vi "VI Tree - error.vi"   [LabVIEW 2020]
uses:
  Filter Error Codes/Filter Error Codes (Array).vi
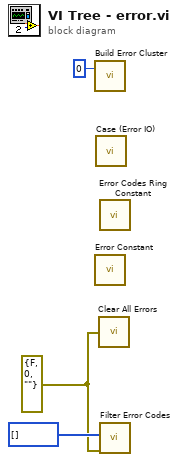
[diagram p0: block diagram]
diagram:
  w1 = errorcluster {"status"=FALSE, "code"=0, "source"=""} ("error in")
  n1 = call "Build Error Cluster.vi"("code"=0) -> ()  [unwired: 1 in, 1 out]
  n2 = call "Error Constant.vi"() -> ()  [unwired: 1 in]
  n3 = call "Case (Error IO).vi"() -> ()  [unwired: 1 in]
  n4 = call "Clear All Errors.vi"("Error In"=w1) -> ()  [unwired: 3 in, 1 out]
  n5 = call "Error Codes Ring Constant.vi"() -> ()  [unwired: 1 in]
  n6 = call-poly "Filter Error Codes.vi"("Error In"=w1, "Error Codes to Filter"=i32[] [] ("error codes to filter")) -> ()  [unwired: 7 in, 3 out]
